vi "Parallel Event Task.vi"(9 "Stop reference":refnum<vi>, 10 "Field Names":string[](array[string]) caption="field names", 11 "map of references":T1(c390)) -> ()   [LabVIEW 2019]
uses:
  PV Info.ctl
  CaLab.lvlib
  Private/CaLabEvent_PV-1D.vi
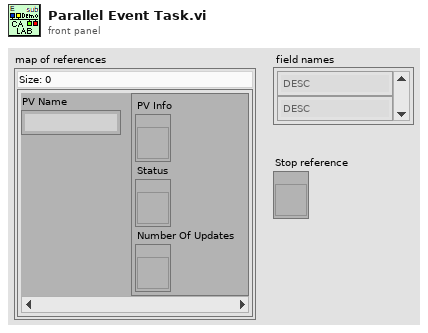
[diagram p1: front panel]
types:
  T1 = map{string, cluster{"PV Info":refnum<vi>, "Status":refnum<vi>, "Number Of Updates":refnum<vi>}}
  T2 = typedef "CaLab.lvlib/PV Info.ctl" = cluster{"Name":string, "Elements":i32, "Values (string)":string[], "Values (number)":dbl[], "Status (string)":string, "Status (number)":i16, "Severity (string)":string, "Severity (number)":i16, "Timestamp (string)":string, "Timestamp (number)":i32, "Field Names":string[], "Field Values":string[], "Error":errorcluster}
  T3 = cluster{"PV Info":refnum<vi>, "Status":refnum<vi>, "Number Of Updates":refnum<vi>}
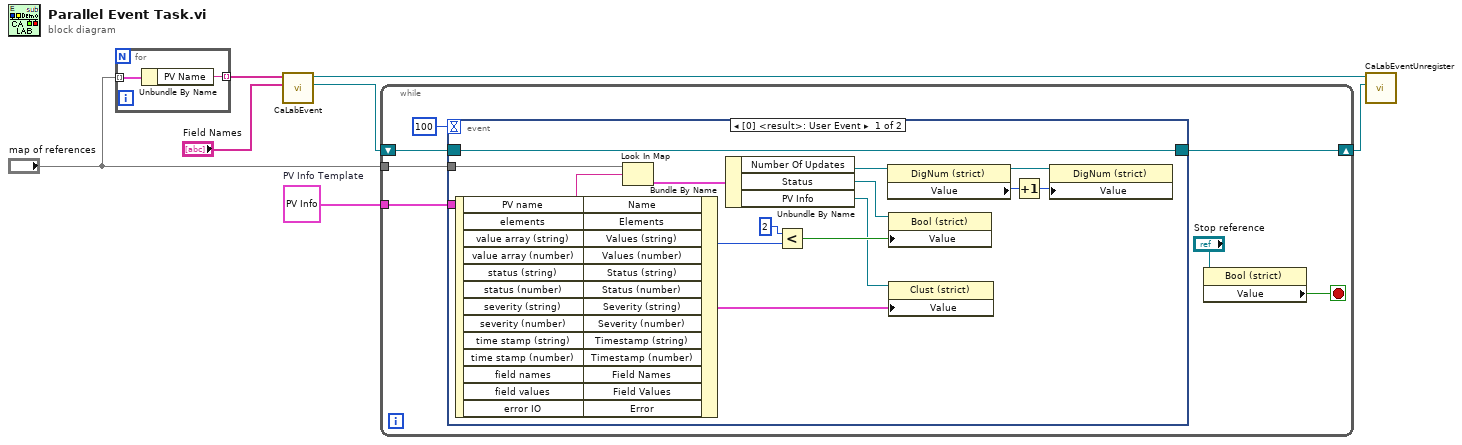
[diagram p0: block diagram]
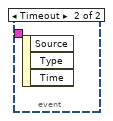
[diagram p2: hidden frame]
diagram:
  w6 = T2 {"Name"="TestPV:ai1", "Elements"=1, "Values (string)"=["3"], "Values (number)"=[3.0], "Status (string)"="NO_ALARM", "Status (number)"=0, "Severity (string)"="NO_ALARM", "Severity (number)"=0, "Timestamp (string)"="2022-07-21 10:27:19.961173", "Timestamp (number)"=1027240039, "Field Names"=[], "Field Values"=[], "Error"={"status"=FALSE, "code"=0, "source"="Normal successful completion"}}  # PV Info Template
  n1 = for {
    tunnel: "map of references" -> [w9] mode=indexing
    tunnel: [w8] -> w3 mode=indexing
    n2 = Unbundle By Name(w9) -> ("PV Name"=w8:string)
  }
  n3 = call-poly "CaLabEvent.vi"("Field Names"="Field Names", "PV Names"=w3) -> ("Refnum"=w7:refnum<event-registration>, "Event"=w4:refnum<user-event>)  [unwired: 6 in, 2 out]
  n4 = while {
    tunnel: "map of references" -> [w15]
    tunnel: w6 -> [w14]
    shift-right: [w13] -> w5
    shift-left: w7 -> [w16]
    stop <- w10 stop-if-true
    n5 = event shown="[0] <result>: User Event" {
      selector: w16 -> [w23 _]
      dyn-events: [w23 _] -> w13
      timeout: 100 -> [_ _]
      tunnel: w15 -> [w42 _]
      tunnel: w14 -> [w25 _]
      event User Event {
        n6 = event-data() -> ("PV name"=w21:string, "elements"=w37:i32, "value array (string)"=w36:string[], "value array (number)"=w35:dbl[], "status (string)"=w34:string, "status (number)"=w33:i16, "severity (string)"=w32:string, "severity (number)"=w31:i16, "time stamp (string)"=w30:string, "time stamp (number)"=w29:i32, "field names"=w28:string[], "field values"=w27:string[], "error IO"=w26:errorcluster)  [unwired: 1 in]
        n7 = Bundle By Name(cluster=w25, "Name"=w21, "Elements"=w37, "Values (string)"=w36, "Values (number)"=w35, "Status (string)"=w34, "Status (number)"=w33, "Severity (string)"=w32, "Severity (number)"=w31, "Timestamp (string)"=w30, "Timestamp (number)"=w29, "Field Names"=w28, "Field Values"=w27, "Error"=w26) -> (w24:T2)
        n8 = Look In Map(map=w42, key=w21) -> (value=w20:T3)  [unwired: 1 in, 1 out]
        n9 = Unbundle By Name(w20) -> ("Number Of Updates"=w19:refnum<vi>, "Status"=w18:refnum<vi>, "PV Info"=w17:refnum<vi>)
        n10 = Less?(x=i16 2, y=w31) -> (x < y?=w39:bool)
        n11 = property class="DigNum (strict)"(reference=w19) -> (reference out=w38:refnum<vi>, "Value"=w22:i32)  [unwired: 1 in, 1 out]
        n12 = property class="Bool (strict)"(reference=w18, "Value"=w39) -> ()  [unwired: 1 in, 2 out]
        n13 = property class="Clust (strict)"(reference=w17, "Value"=w24) -> ()  [unwired: 1 in, 2 out]
        n14 = Increment(x=w22) -> (x+1=w41:i32)
        n15 = property class="DigNum (strict)"(reference=w38, "Value"=w41) -> ()  [unwired: 1 in, 2 out]
      }
      event Timeout {
        n16 = event-data() -> ()  [unwired: 1 in, 3 out]
      }
    }
    n17 = property class="Bool (strict)"(reference="Stop reference") -> ("Value"=w10:bool)  [unwired: 1 in, 2 out]
  }
  n18 = call "CaLabEventUnregister.vi"("Refnum"=w5, "Event"=w4) -> ()  [unwired: 9 in, 1 out]
